vi "WaitInput.vi"(6 "time(0.1)":i32=100, 7 "Enum":T1, 8 "error in (no error)":errorcluster, 9 "Wait?":bool=TRUE, 10 "Status":bool) -> (0 "error out":errorcluster, 1 "TimeOut":bool, 2 "StatusOut":bool)   [LabVIEW 2019, in "Station Action.lvclass"]
uses:
  Station Action.lvclass
  Ctrl/S2 Station Input.ctl
  LLB/Commonly VI/Main Glb.vi
  LLB/Commonly VI.lvlib
panel:
  in  "Boolean":bool=TRUE
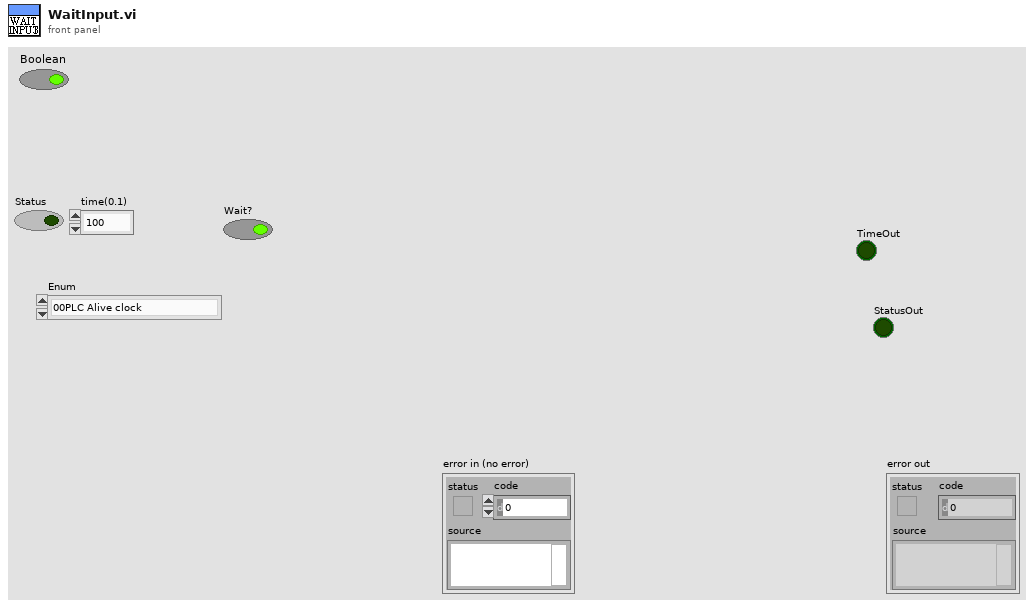
[diagram p1: front panel]
types:
  T1 = typedef "S2 Station Input.ctl" = enum16{"00PLC Alive clock", "01PLC狀態(手動)", "02PLC狀態(自動)", "03PLC Alarm", "04備用", "05備用", "06備用", "07備用", "08備用", "09備用", "10載盤有料for條碼", "11_備用", "12_備用", "13_備用", "14_備用", "15_備用", "16_備用", "17_備用", "18_備用", "19_備用", "20_載盤有料訊號ForS2站", "21_PLC下達可測電流訊號", "22_PLC下達可測電壓訊號"}
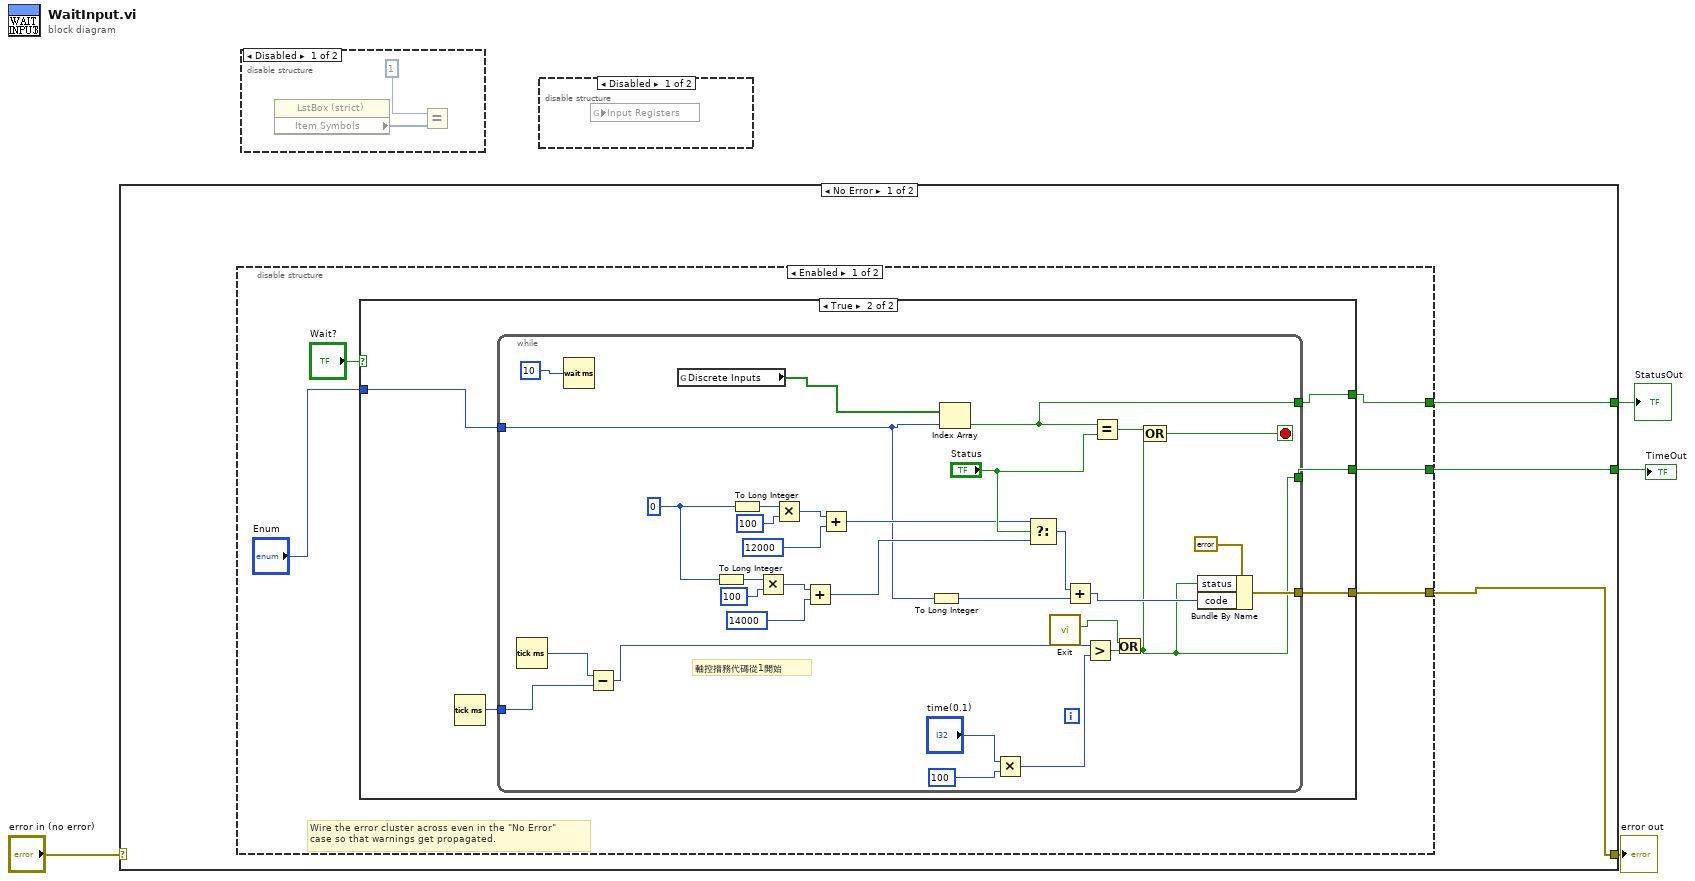
[diagram p0: block diagram]
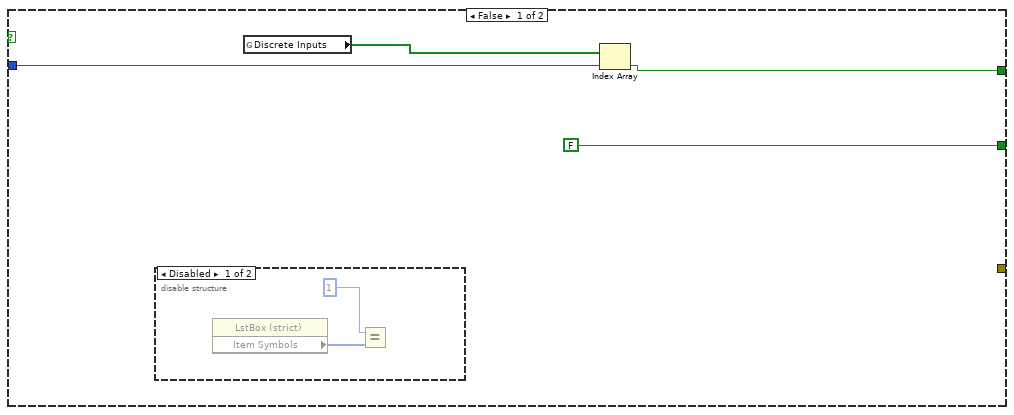
[diagram p4: hidden frame]
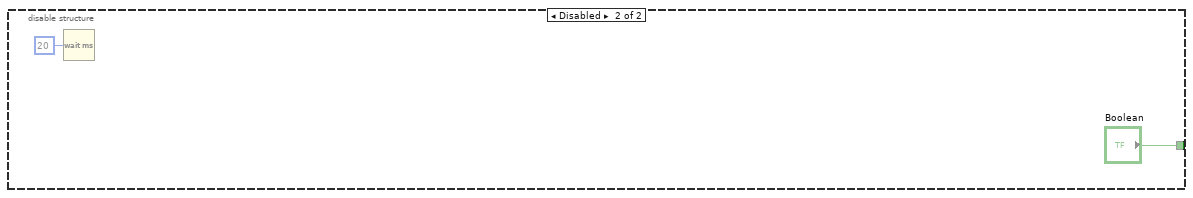
[diagram p6: hidden frame]
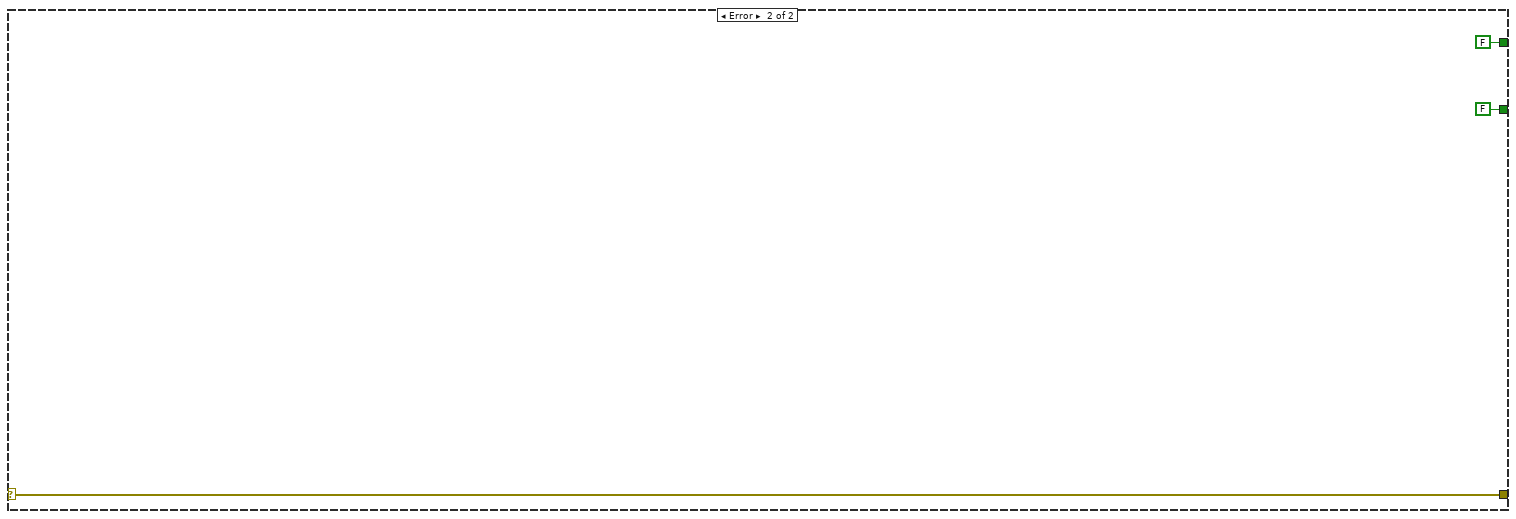
[diagram p7: hidden frame]
diagram:
  n1 = case shown="No Error" "error in (no error)" {
    selector: "error in (no error)" -> [_ w60]
    tunnel: [w7 w60] -> w3
    tunnel: [w6 FALSE] -> w2
    tunnel: [w5 FALSE] -> w1
    frame No Error {
      n2 = disable-structure shown="Enabled" {
        disable-tunnel: [w11 _] -> w7
        disable-tunnel: [w10 _] -> w6
        disable-tunnel: [w9 "Boolean"] -> w5
        frame Enabled {
          # "Wire the error cluster across even in the \"No Error\"\ncase so that warnings get propagated."
          n3 = case shown="True" "Wait?" {
            tunnel: [FALSE w23] -> w10
            tunnel: [_ w22] -> w11
            tunnel: [w16 w21] -> w9
            tunnel: "Enum" -> [w13 w19]
            frame False {
              n4 = disable-structure shown="Disabled" {
                frame Disabled {
                  n5 = property class="LstBox (strict)"() -> ("Item Symbols"=w17:i32[])  [unwired: 2 in, 2 out]
                  n6 = Equal?(x=1, y=w17) -> ()  [unwired: 1 out]
                }
                frame Enabled {
                }
              }
              n7 = global read "Main Glb.vi" "Discrete Inputs"() -> (w14:bool[])
              n8 = Index Array(array=w14, index=w13) -> (element=w16:bool)
            }
            frame True {
              n9 = Tick Count (ms)() -> (millisecond timer value=w20:u32)
              n10 = while {
                tunnel: [w46] -> w23
                tunnel: [w50] -> w22
                tunnel: [w29] -> w21
                tunnel: w20 -> [w31]
                tunnel: w19 -> [w24]
                stop <- w54 stop-if-true
                w25 = 0 ("number")
                # "軸控措務代碼從1開始"
                n11 = Tick Count (ms)() -> (millisecond timer value=w32:u32)
                n12 = Wait (ms)(milliseconds to wait=u32 10) -> ()  [unwired: 1 out]
                n13 = Subtract(x=w32, y=w31) -> (x-y=w30:u32)
                n14 = global read "Main Glb.vi" "Discrete Inputs"() -> (w26:bool[])
                n15 = To Long Integer(number=w25) -> (32bit integer=w37:i32)
                n16 = To Long Integer(number=w25) -> (32bit integer=w45:i32)
                n17 = Multiply(x=w37, y=100) -> (x*y=w39:i32)
                n18 = Multiply(x=w45, y=100) -> (x*y=w43:i32)
                n19 = Add(x=w39, y=14000) -> (x+y=w36:i32)
                n20 = Add(x=w43, y=12000) -> (x+y=w41:i32)
                n21 = To Long Integer(number=w24) -> (32bit integer=w47:i32)
                n22 = Index Array(array=w26, index=w24) -> (element=w29:bool)
                n23 = Multiply(x="time(0.1)", y=u32 100 ("milliseconds to wait")) -> (x*y=w33:u32)
                n24 = Select(t=w41, s="Status", f=w36) -> (s? t:f=w48:i32)
                n25 = call "Exit.vi"() -> ("ExitOut"=w28:bool)  [unwired: 11 in]
                n26 = Add(x=w48, y=w47) -> (x+y=w51:i32)
                n27 = Greater?(x=w30, y=w33) -> (0:w52:bool)
                n28 = Equal?(x=w29, y="Status") -> (x = y?=w53:bool)
                n29 = Or(x=w28, y=w52) -> (x .or. y?=w46:bool)
                n30 = Compound Arithmetic op=OR(w53, w46) -> (w54:bool)
                n31 = Bundle By Name(cluster=errorcluster {"status"=FALSE, "code"=0, "source"=""} ("error Out"), "status"=w46, "code"=w51) -> (w50:errorcluster)
              }
            }
          }
        }
        frame Disabled {
          n32 = Wait (ms)(milliseconds to wait=u32 20) -> ()  [unwired: 1 out]
        }
      }
    }
    frame Error {
    }
  }
  "error out" <- w3
  "TimeOut" <- w2
  "StatusOut" <- w1
  n33 = disable-structure shown="Disabled" {
    frame Disabled {
      n34 = property class="LstBox (strict)"() -> ("Item Symbols"=w61:i32[])  [unwired: 2 in, 2 out]
      n35 = Equal?(x=1, y=w61) -> ()  [unwired: 1 out]
    }
    frame Enabled {
    }
  }
  n36 = disable-structure shown="Disabled" {
    frame Disabled {
      n37 = global read "Main Glb.vi" "Input Registers"() -> ()  [unwired: 1 in]
    }
    frame Enabled {
    }
  }
